vi "Configure AC Bandwidth [AC] Core.vi"(8 "error in (no error)":errorcluster, 9 "ac max frequency (300.0E+3 Hz)":dbl=300000.0 format="%^.2e", 10 "ac min frequency (20.0 Hz)":dbl=20.0 format="%^.2e", 11 "IVI_DMM in":refnum<class "IVI_DMM.lvclass">) -> (0 "error out":errorcluster, 3 "IVI_DMM out":refnum<class "IVI_DMM.lvclass">)   [LabVIEW 2013, in "IVI_DMM.lvlib" / "IVI_DMM.lvclass"]
doc: "This VI configures the AC minimum and maximum frequency for DMMs that take AC voltage or AC current measurements.\n\nThis VI affects the behavior of the instrument only if the IviDmm>Basic Operation>Function property is set to an AC voltage or AC current measurement.\n\nNote:\n\n(1) This VI is part of the IviDmmACMeasurement [AC] extension group."
uses:
  IVI_DMM.lvclass
  IVI_DMM.lvclass/IVI_DMM.ctl
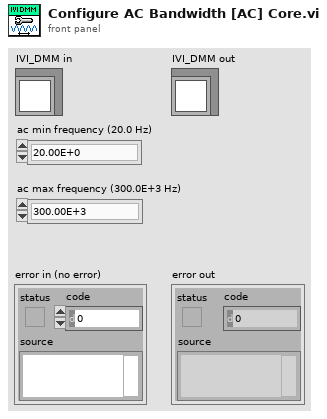
[diagram p1: front panel]
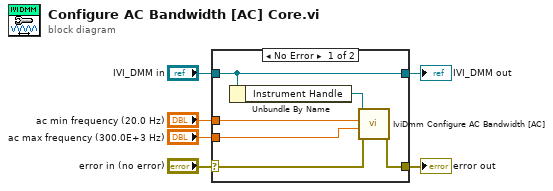
[diagram p0: block diagram]
diagram:
  n1 = case shown="No Error" "error in (no error)" {
    selector: "error in (no error)" -> [w7 w14]
    tunnel: [w8 w14] -> w5
    tunnel: [w12 w13] -> w3
    tunnel: "IVI_DMM in" -> [w12 w13]
    tunnel: "ac min frequency (20.0 Hz)" -> [w10 _]
    tunnel: "ac max frequency (300.0E+3 Hz)" -> [w9 _]
    frame No Error {
      n2 = Unbundle By Name(w12) -> ("Instrument Handle"=w11:refnum<k15>)
      n3 = call <vilib>:"IviDmm Configure AC Bandwidth [AC].vi"("error in (no error)"=w7, "ac max frequency (300.0E+3 Hz)"=w9, "ac min frequency (20.0 Hz)"=w10, "instrument handle"=w11) -> ("error out"=w8:errorcluster)  [unwired: 6 in, 1 out]
    }
    frame Error {
    }
  }
  "error out" <- w5
  "IVI_DMM out" <- w3
